vi "SMO.LaunchDependency.vi"(6 "Shared Resource":bool, 7 "Level":string, 8 "error in (no error)":errorcluster, 9 "Dependency Name":string, 10 "Dependency Type":refnum<class "SMO.lvclass">, 11 "SMO in":refnum<class "SMO.lvclass">) -> (0 "error out":errorcluster, 1 "Unique Name":string, 2 "Dependency Reference":refnum<class "SMO.lvclass">, 3 "SMO out":refnum<class "SMO.lvclass">)   [LabVIEW 2013, in "SMO.lvclass"]
uses:
  SMO.lvclass
  SMO.lvclass/SMO.ctl
  Support/Attribute.Owner/Attribute.Owner.lvclass/Attribute.Owner.ctl
  GetVariant(Attr).vi
  ReftoDVR--SMO.vi
  Support/Attribute.Owner/Attribute.Owner.lvclass
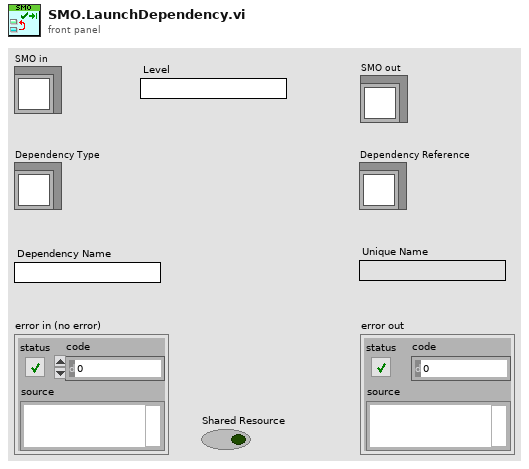
[diagram p1: front panel]
types:
  T1 = typedef "SMO.lvclass/ProcessRegistrationRefnum.ctl" = refnum<event-registration>
  T2 = typedef "SMO.lvclass/Public Events.ctl" = cluster{"Error":refnum<user-event>, "State":refnum<user-event>, "Reserve State":refnum<user-event>}
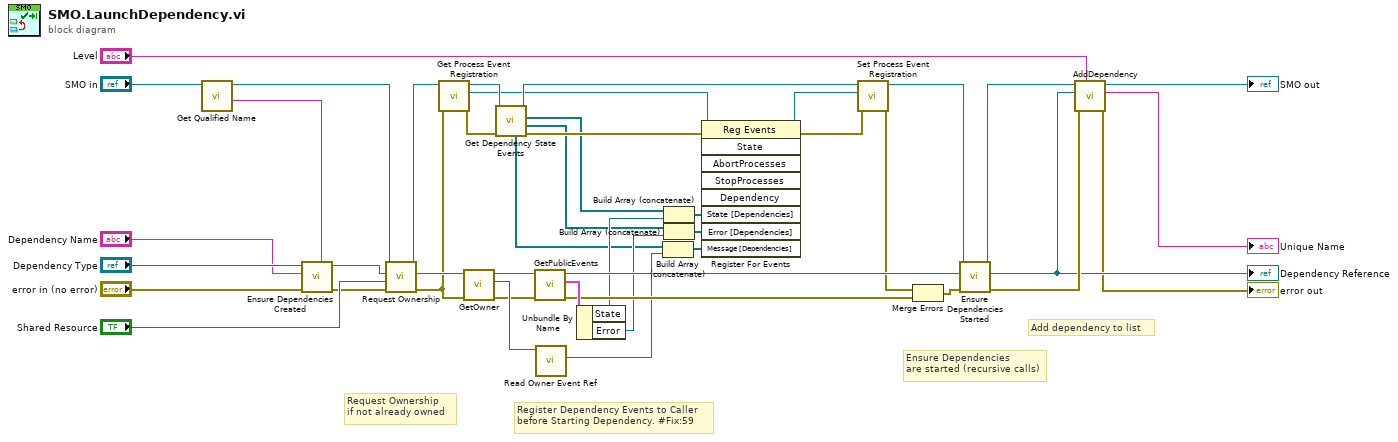
[diagram p0: block diagram]
diagram:
  # "Register Dependency Events to Caller\nbefore Starting Dependency. #Fix:59"
  # "Add dependency to list"
  # "Ensure Dependencies\nare started (recursive calls)"
  # "Request Ownership\nif not already owned"
  n1 = call "Get Qualified Name.vi"("SMO"="SMO in") -> ("Reserved Qualified Name"=w29:string, "SMO out"=w30:refnum<class "SMO.lvclass">)  [unwired: 7 in, 2 out]
  n2 = call "Ensure Dependencies Created.vi"("Owner Qualified Name"=w29, "error in (no error)"="error in (no error)", "Dependency Name"="Dependency Name", "SMO in"="Dependency Type") -> ("error out"=w39:errorcluster, "SMO out"=w43:refnum<class "SMO.lvclass">)  [unwired: 5 in, 1 out]
  n3 = call "Request Ownership.vi"("error in (no error)"=w39, "Shared Resource"="Shared Resource", "Dependency"=w43, "SMO in"=w30) -> ("error out"=w12:errorcluster, "Dependency out"=w16:refnum<class "SMO.lvclass">, "SMO out"=w28:refnum<class "SMO.lvclass">)  [unwired: 5 in]
  n4 = call "Get Process Event Registration.vi"("error in (no error)"=w12, "SMO in"=w28) -> ("error out"=w24:errorcluster, "Event Registration Refnum"=w21:T1, "SMO out"=w26:refnum<class "SMO.lvclass">)  [unwired: 7 in]
  n5 = call "GetOwner.vi"("error in (no error)"=w12, "SMO in"=w16) -> ("error out"=w13:errorcluster, "Owner"=w17:refnum<class "Attribute.Owner.lvclass">, "SMO out"=w18:refnum<class "SMO.lvclass">)  [unwired: 6 in, 1 out]
  n6 = call "Get Dependency State Events.vi"("error in (no error)"=w24, "SMO in"=w26) -> ("error out"=w23:errorcluster, "Error [Dependencies]"=w5:refnum<user-event>[], "State [Dependencies]"=w8:refnum<user-event>[], "SMO out"=w25:refnum<class "SMO.lvclass">, "Message [Dependencies]"=w2:refnum<user-event>[])  [unwired: 4 in, 1 out]
  n7 = call "GetPublicEvents.vi"("error in (no error)"=w13, "SMO"=w18) -> ("error out"=w14:errorcluster, "Public Events"=w19:T2, "SMO out"=w15:refnum<class "SMO.lvclass">)  [unwired: 7 in]
  n8 = call "Read Owner Event Ref.vi"("Attribute.Owner in"=w17) -> ("Upstream Ref"=w3:refnum<user-event>)  [unwired: 8 in, 2 out]
  n9 = Unbundle By Name(w19) -> ("State"=w9:refnum<user-event>, "Error"=w6:refnum<user-event>)
  n10 = Build Array (concatenate)(w2, w3) -> (w1:refnum<user-event>[])
  n11 = Build Array (concatenate)(w8, w9) -> (w7:refnum<user-event>[])
  n12 = Build Array (concatenate)(w5, w6) -> (w4:refnum<user-event>[])
  n13 = register-events(reference=w21, error in=w23, w7, w4, w1) -> (reference out=w20:T1, error out=w22:errorcluster)  [unwired: 4 in]
  n14 = call "Set Process Event Registration.vi"("error in (no error)"=w22, "Event Registration Refnum"=w20, "SMO in"=w25) -> ("error out"=w11:errorcluster, "SMO out"=w27:refnum<class "SMO.lvclass">)  [unwired: 7 in]
  n15 = Merge Errors(w11, w14) -> (w10:errorcluster)
  n16 = call "Ensure Dependencies Started.vi"("error in (no error)"=w10, "Dependency in"=w15, "SMO in"=w27) -> ("error out"=w36:errorcluster, "Started Dependency"=w35:refnum<class "SMO.lvclass">, "SMO out"=w37:refnum<class "SMO.lvclass">)  [unwired: 6 in]
  "Dependency Reference" <- w35
  n17 = call "AddDependency.vi"("Level"="Level", "error in (no error)"=w36, "Dependency"=w35, "SMO in"=w37) -> ("error out"=→"error out":errorcluster, "Unique Name"=→"Unique Name":string, "SMO out"=→"SMO out":refnum<class "SMO.lvclass">)  [unwired: 5 in]
